vi "geneXY.vi"() -> ()   [LabVIEW 2013]
uses:
  <vilib>/Analysis/Matrix/Datatypes/RealMatrix.ctl
  <vilib>/Analysis/Matrix/NI_Matrix.lvlib
panel:
  out "final XY":T1
  in  "Number of Positions":u32=40
  in  "Spacing Y":dbl=0.1
  in  "Spacing X":dbl=0.1
  in  "Method":u8(ring) items=["Spiral Scan", "Column Scan", "Line Scan"]
  out "Field\nHeigth (mm)":dbl
  out "Field\nWidth (mm)":dbl
  in  "Microscope Objective\nMagnification":dbl=60.0 min=1.0 max=1000.0 step=1.0
  # "mm"
  # "X"
  # "mm"
  # "mm"
  # "mm"
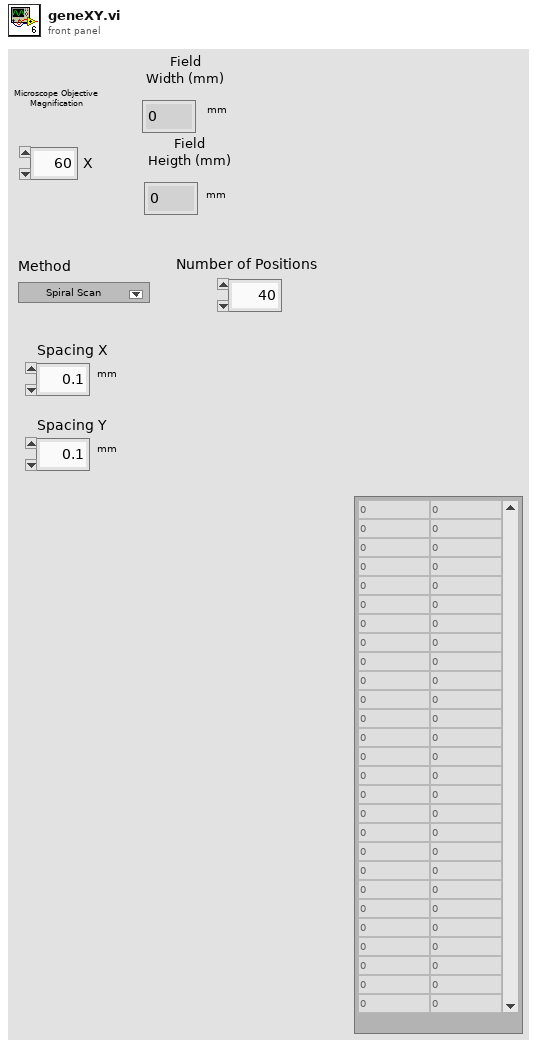
[diagram p1: front panel]
types:
  T1 = typedef "NI_Matrix.lvlib/RealMatrix.ctl" = dbl[][]
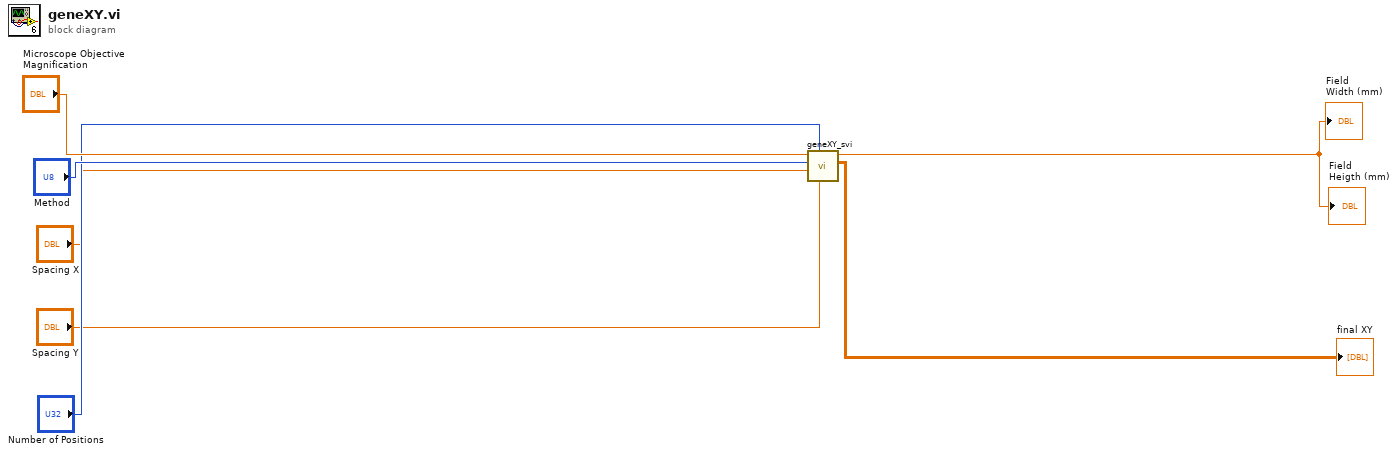
[diagram p0: block diagram]
diagram:
  n1 = call "geneXY_svi.vi"("Spacing Y"="Spacing Y", "Number of Positions"="Number of Positions", "Spacing X"="Spacing X", "Method"="Method", "Microscope Objective\nMagnification"="Microscope Objective\nMagnification") -> ("Real Matrix"=→"final XY":T1, "Numérique"=→"Field\nWidth (mm)" →"Field\nHeigth (mm)":dbl)  [unwired: 5 in]
